vi "Executable Path To Command Line String.vi"(10 "Executable Path":path) -> (2 "System Exec String":string)   [LabVIEW 2017]
doc: "Given the path to an executable, returns the correct string to pass to System Exec VI to be able to run the executable. This does little on Linux and Windows, but on Mac, where applications can be folders, this VI will determine the path to the binary of the executable."
uses:
  <vilib>/regexp/Match Regular Expression.xnode
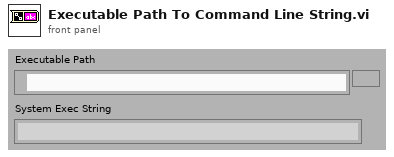
[diagram p1: front panel]
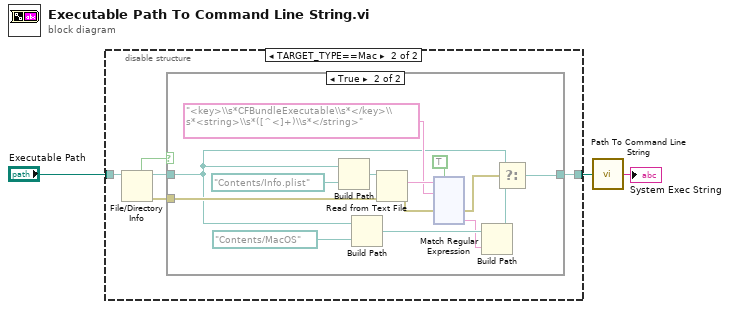
[diagram p0: block diagram]
diagram:
  n1 = disable-structure shown="TARGET_TYPE==Mac" {
    disable-tunnel: [w4 w6] -> w2
    disable-tunnel: "Executable Path" -> [w4 w9]
    frame condition #0 (active) {
    }
    frame condition #1 {
      n2 = File/Directory Info(path=w9) -> (path out=w7:path, directory=w8:bool, error out=w5:errorcluster)  [unwired: 1 in, 4 out]
      n3 = case shown="True" w8 {
        tunnel: w7 -> [w10 w14]
        tunnel: [w10 w12] -> w6
        tunnel: w5 -> [_ w21]
        frame False {
        }
        frame True {
          n4 = Build Path(base path=w14, name or relative path=path "Contents/Info.plist" ("path out")) -> (appended path=w22:path)
          n5 = Build Path(base path=w14, name or relative path=path "Contents/MacOS" ("path out")) -> (appended path=w17:path)
          n6 = Read from Text File(file (use dialog)=w22, error in=w21) -> (text=w19:string, error out=w20:errorcluster)  [unwired: 4 out]
          n7 = xnode "Match Regular Expression"("input string"=w19, "regular expression"="<key>\\s*CFBundleExecutable\\s*</key>\\s*<string>\\s*([^<]+)\\s*</string>", "error in"=w20, "ignore case? (F)"=TRUE) -> ("error out"=w15:errorcluster, "submatch 1"=w16:string)  [unwired: 1 in, 5 out]
          n8 = Build Path(base path=w17, name or relative path=w16) -> (appended path=w13:path)
          n9 = Select(t=w14, s=w15, f=w13) -> (s? t:f=w12:path)
        }
      }
    }
  }
  n10 = call <vilib>:"Path To Command Line String.vi"("path"=w2) -> ("string"=→"System Exec String":string)
